vi "vi.vi"() -> ()   [LabVIEW 2021]
uses:
  <vilib>/DAQmx/read.llb/DAQmx Read (Analog 1D Wfm NChan NSamp).vi
  <vilib>/DAQmx/create/channels.llb/DAQmx Create Channel (AI-Voltage-Basic).vi
  <vilib>/DAQmx/configure/timing.llb/DAQmx Timing (Sample Clock).vi
  <vilib>/DAQmx/miscellaneous.llb/DAQmx Fill In Error Info.vi
panel:
  out "task out":refnum<k21>
  out "Waveform Chart":waveform(dbl)[](graph)
  out "task done? AI":bool
  in  "stop":bool
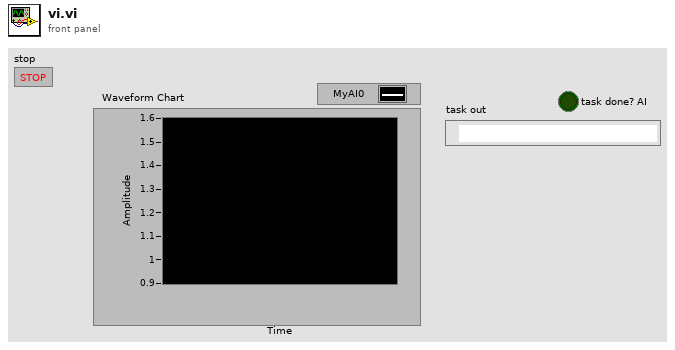
[diagram p1: front panel]
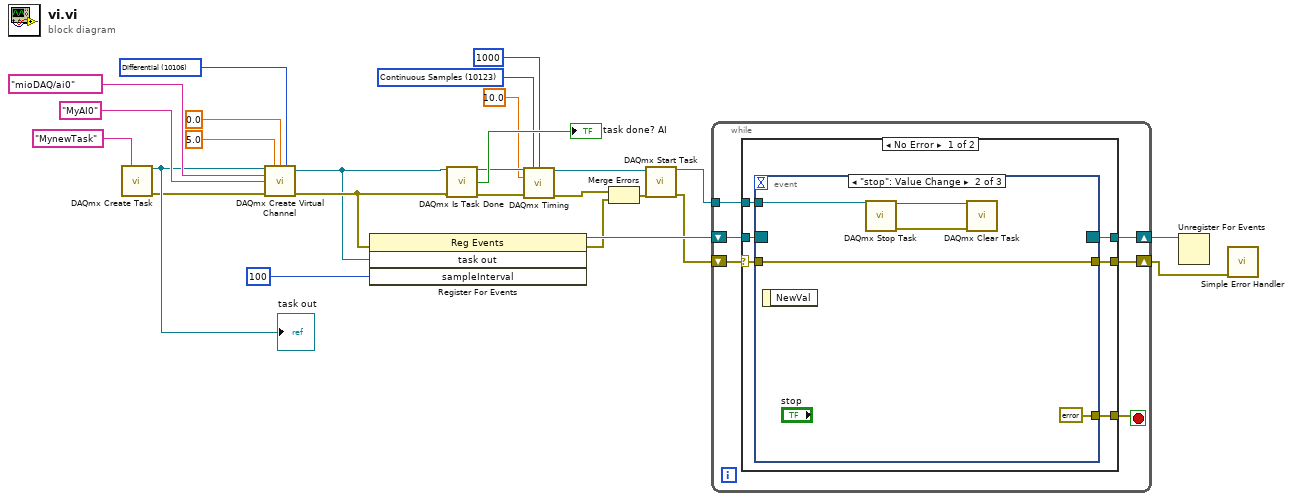
[diagram p0: block diagram]
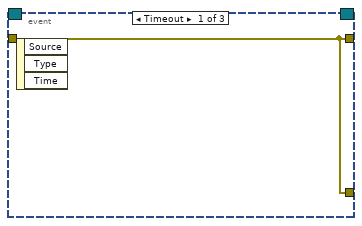
[diagram p2: hidden frame]
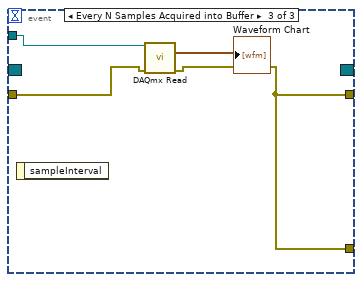
[diagram p3: hidden frame]
diagram:
  w21 = 10106 items=["Default"=-1, "RSE"=10083, "NRSE"=10078, "Differential"=10106, "Pseudodifferential"=12529] ("input terminal configuration")
  w16 = 10123 items=["Finite Samples"=10178, "Continuous Samples"=10123, "Hardware Timed Single Point"=12522] ("sample mode")
  n1 = call <vilib>:"DAQmx Create Task.vi"("new task name"="MynewTask") -> ("task out"=w4:refnum<k21>, "error out"=w3:errorcluster)  [unwired: 13 in]
  "task out" <- w4
  n2 = call-poly <vilib>:"DAQmx Create Virtual Channel.vi"("task in"=w4, "maximum value"=5.0, "minimum value"=0.0, "input terminal configuration"=w21, "physical channels"=tag "mioDAQ/ai0", "name to assign"="MyAI0" ("new task name"), "error in"=w3) -> ("task out"=w1:refnum<k21>, "error out"=w2:errorcluster)  [unwired: 7 in]
  n3 = register-events(error in=w2, w1, u32 100 ("sampleInterval")) -> (reference out=w26:refnum<event-registration>, error out=w14:errorcluster)  [unwired: 1 in]
  n4 = call <vilib>:"DAQmx Is Task Done.vi"("task/channels in"=w1, "error in"=w2) -> ("task out"=w23:refnum<k21>, "task done?"=→"task done? AI":bool, "error out"=w22:errorcluster)  [unwired: 11 in]
  n5 = call-poly <vilib>:"DAQmx Timing.vi"("task/channels in"=w23, "sample mode"=w16, "samples per channel"=1000, "rate"=10.0, "error in"=w22) -> ("task out"=w12:refnum<k21>, "error out"=w13:errorcluster)  [unwired: 9 in]
  n6 = Merge Errors(w13, w14) -> (w15:errorcluster)
  n7 = call <vilib>:"DAQmx Start Task.vi"("task/channels in"=w12, "error in"=w15) -> ("task out"=w10:refnum<k21>, "error out"=w11:errorcluster)  [unwired: 12 in]
  n8 = while {
    tunnel: w10 -> [w27]
    shift-right: [w29] -> w5
    shift-left: w11 -> [w30]
    shift-right: [w31] -> w25
    shift-left: w26 -> [w32]
    stop <- w28 stop-if-true
    n9 = case shown="No Error" w30 {
      selector: w30 -> [w36 w49]
      tunnel: w32 -> [w38 w50]
      tunnel: [w37 w50] -> w31
      tunnel: [w35 _] -> w29
      tunnel: [w34 w49] -> w28
      tunnel: w27 -> [w33 _]
      frame No Error {
        n10 = event shown="[1] \"stop\": Value Change" {
          selector: w38 -> [_ _ _]
          dyn-events: [_ _ _] -> w37
          timeout: _ -> [_ _ _]
          tunnel: w36 -> [w39 w40 w47]
          tunnel: [w39 w40 w46] -> w35
          tunnel: [w39 errorcluster {"status"=TRUE, "code"=0, "source"=""} ("error out") w46] -> w34
          tunnel: w33 -> [_ w41 w48]
          event Timeout {
            n11 = event-data() -> ()  [unwired: 1 in, 3 out]
          }
          event "stop": Value Change {
            n12 = event-data() -> ()  [unwired: 1 in, 1 out]
            n13 = call <vilib>:"DAQmx Stop Task.vi"("task/channels in"=w41) -> ("task out"=w42:refnum<k21>, "error out"=w43:errorcluster)  [unwired: 13 in]
            n14 = call <vilib>:"DAQmx Clear Task.vi"("task in"=w42, "error in"=w43) -> ()  [unwired: 13 in, 1 out]
          }
          event Every N Samples Acquired into Buffer {
            n15 = event-data() -> ()  [unwired: 1 in, 1 out]
            n16 = call-poly <vilib>:"DAQmx Read.vi"("task/channels in"=w48, "error in"=w47) -> ("data"=→"Waveform Chart":waveform(dbl)[], "error out"=w46:errorcluster)  [unwired: 11 in, 1 out]
          }
        }
      }
      frame Error {
      }
    }
  }
  n17 = Unregister For Events(event registration refnum=w25) -> ()  [unwired: 1 in, 1 out]
  n18 = call <vilib>:"Simple Error Handler.vi"("error in (no error)"=w5) -> ()  [unwired: 4 in, 5 out]
